vi "Thev-Optimization Function.vi"(3 "output control":T1, 4 "data":variant, 5 "X":dbl[](array[numeric]), 6 "a":dbl[](array[numeric])) -> (0 "error out":errorcluster, 1 "f'(X,a)":dbl[][](array[numeric]), 2 "f(X,a)":dbl[](array[numeric]))   [LabVIEW 2015]
doc: "This template is the starting point for creating a model function to be passed to the Nonlinear Curve Fit.vi."
uses:
  <vilib>/gmath/NumericalOptimization/LM_output select.ctl
  <vilib>/gmath/NI_Gmath.lvlib
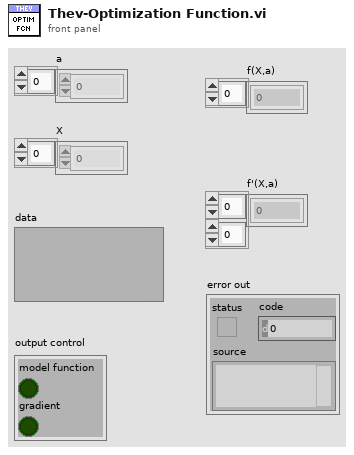
[diagram p1: front panel]
types:
  T1 = typedef "NI_Gmath.lvlib/LM_output select.ctl" = cluster{"model function":bool, "gradient":bool}
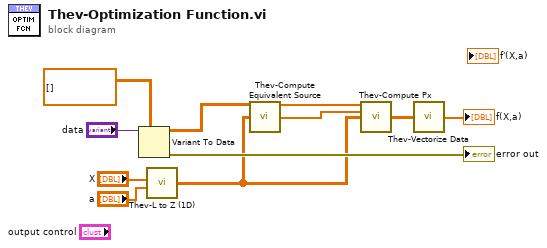
[diagram p0: block diagram]
diagram:
  n1 = Variant To Data(type=cdb[][] [], Variant="data") -> (data=w6:cdb[][], error out=→"error out":errorcluster)  [unwired: 1 in]
  n2 = call "Thev-L to Z (1D).vi"("L (mm)"="a", "Frequency (Hz)"="X") -> ("Zx"=w3:cdb[][])  [unwired: 2 in]
  n3 = call "Thev-Compute Equivalent Source.vi"("Px"=w6, "Zx"=w3) -> ("Ps"=w5:cdb[], "Zs"=w4:cdb[])  [unwired: 12 in]
  n4 = call "Thev-Compute Px.vi"("Ps"=w5, "Zs"=w4, "Zx"=w3) -> ("Px"=w1:cdb[][])  [unwired: 12 in]
  n5 = call "Thev-Vectorize Data.vi"("2D CDB"=w1) -> ("1D DBL"=→"f(X,a)":dbl[])  [unwired: 14 in]
